vi "get horizontal angle.vi"(10 "Point 2":cluster{"X":sgl, "Y":sgl}, 11 "Point 1":cluster{"X":sgl, "Y":sgl}) -> (3 "Angle w.r.t horizontal\n(in degrees)":sgl)   [LabVIEW 2019]
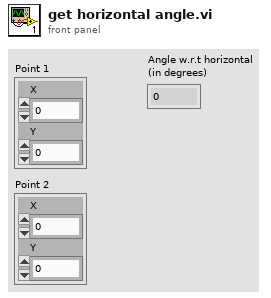
[diagram p1: front panel]
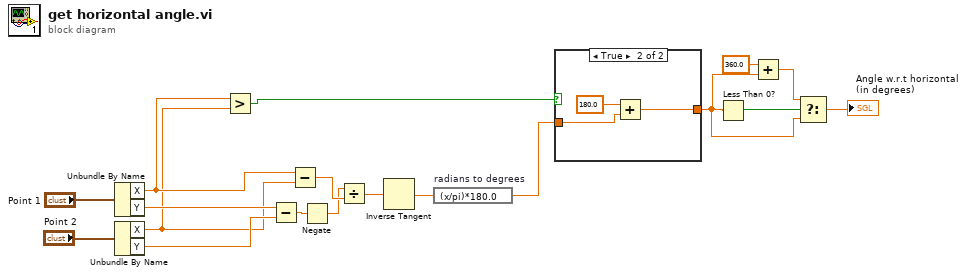
[diagram p0: block diagram]
diagram:
  n1 = Unbundle By Name("Point 1") -> ("X"=w11:sgl, "Y"=w16:sgl)
  n2 = Unbundle By Name("Point 2") -> ("X"=w10:sgl, "Y"=w15:sgl)
  n3 = Greater?(x=w11, y=w10) -> (0:w9:bool)
  n4 = Subtract(x=w16, y=w15) -> (x-y=w7:sgl)
  n5 = Subtract(x=w11, y=w10) -> (x-y=w14:sgl)
  n6 = Negate(x=w7) -> (-x=w6:sgl)
  n7 = Divide(x=w6, y=w14) -> (x/y=w13:sgl)
  n8 = Inverse Tangent(1:w13) -> (0:w12:sgl)
  n9 = expression code="(x/pi)*180.0" "radians to degrees"(w12) -> (w8:sgl)
  n10 = case shown="True" w9 {
    tunnel: w8 -> [w19 w22]
    tunnel: [w19 w20] -> w2
    frame False {
    }
    frame True {
      n11 = Add(x=sgl 180.0, y=w22) -> (x+y=w20:sgl)
    }
  }
  n12 = Less Than 0?(x=w2) -> (x < 0?=w5:bool)
  n13 = Add(x=sgl 360.0, y=w2) -> (x+y=w3:sgl)
  n14 = Select(t=w3, s=w5, f=w2) -> (s? t:f=→"Angle w.r.t horizontal\n(in degrees)":sgl)
